vi "LLTF_full.vi"() -> ()   [LabVIEW 2019]
panel:
  out "CurrentWavelength":dbl
  out "CurrentAngle":dbl
  out "Device moved":bool
  in  "p_TargetWavelength":dbl
  in  "xphyspecLib.IXPhySpec":refnum<k7>
  out "Detected?":bool
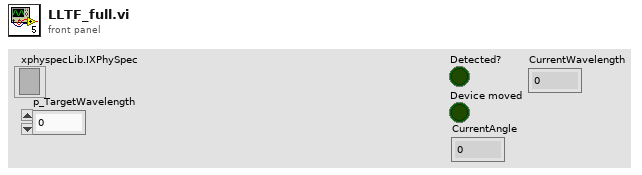
[diagram p1: front panel]
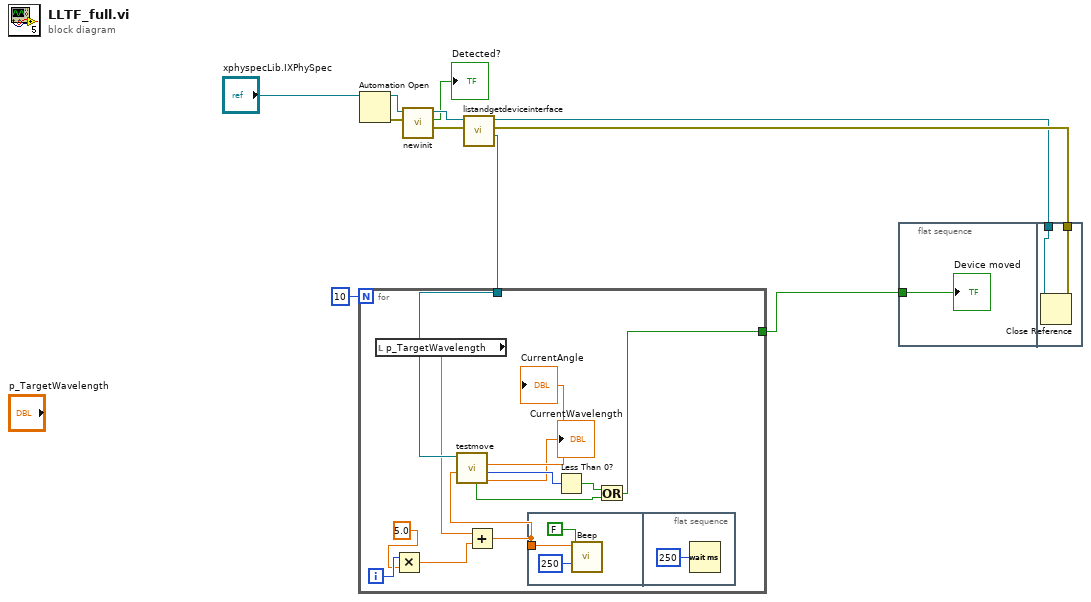
[diagram p0: block diagram]
diagram:
  n1 = Automation Open(Automation Refnum="xphyspecLib.IXPhySpec") -> (Automation Refnum=w7:refnum<k7>, error out=w6:errorcluster)  [unwired: 3 in]
  n2 = call "newinit.vi"("error in"=w6, "Automation Refnum"=w7) -> ("error out"=w10:errorcluster, "Detected?"=→"Detected?":bool, "xphyspecLib.IXPhySpec out"=w11:refnum<k7>)  [unwired: 7 in]
  n3 = call "listandgetdeviceinterface.vi"("error in (no error)"=w10, "reference"=w11) -> ("LLTFDevice Interface"=w5:refnum<k7>, "error out to close"=w3:errorcluster, "reference out to lose"=w2:refnum<k7>)  [unwired: 6 in, 1 out]
  n4 = for {
    N: 10 -> [_]
    tunnel: w5 -> [w23]
    tunnel: [w17] -> w4
    i -> [w16]
    n5 = local read "p_TargetWavelength"() -> (w14:dbl)
    n6 = Multiply(x=w16, y=5.0) -> (x*y=w13:dbl)
    n7 = Add(x=w14, y=w13) -> (x+y=w12:dbl)
    n8 = call "testmove.vi"("p_TargetWavelength"=w12, "reference"=w23) -> ("CurrentWavelength"=→"CurrentWavelength":dbl, "MovetoWavelength"=w22:i32, "CurrentAngle"=→"CurrentAngle":dbl, "Timed Out"=w18:bool)  [unwired: 4 in, 2 out]
    n9 = flat-sequence {
      tunnel: w12 -> [w24]
      frame #0 {
        n10 = call <vilib>:"Beep.vi"("use system alert? (T)"=FALSE, "duration (msec)"=u32 250, "frequency (Hz)"=w24) -> ()  [unwired: 9 in]
      }
      frame #1 {
        n11 = Wait (ms)(milliseconds to wait=u32 250) -> ()  [unwired: 1 out]
      }
    }
    n12 = Less Than 0?(x=w22) -> (x < 0?=w21:bool)
    n13 = Or(x=w21, y=w18) -> (x .or. y?=w17:bool)
  }
  n14 = flat-sequence {
    tunnel: w4 -> [w28]
    tunnel: w3 -> [w30]
    tunnel: w2 -> [w29]
    frame #0 {
      "Device moved" <- w28
    }
    frame #1 {
      n15 = Close Reference(reference=w29, error in (no error)=w30) -> ()  [unwired: 1 out]
    }
  }
